vi "AddCurve.vi"(5 "VarPar":string, 7 "CurveName":string, 8 "error in":errorcluster caption="entrée d'erreur (pas d'erreur)", 9 "Y Array":dbl[](array[numeric]), 10 "X Array":dbl[](array[numeric]), 11 "InterfaceIn":refnum<class "Interface.lvclass">) -> (0 "error out":errorcluster caption="sortie d'erreur", 3 "InterfaceOut":refnum<class "Interface.lvclass">)   [LabVIEW 2019, in "Interface.lvclass"]
uses:
  Interface.lvclass
  AddCurveStates.ctl
  CurveSetup.ctl
  Interface.lvclass/Interface.ctl
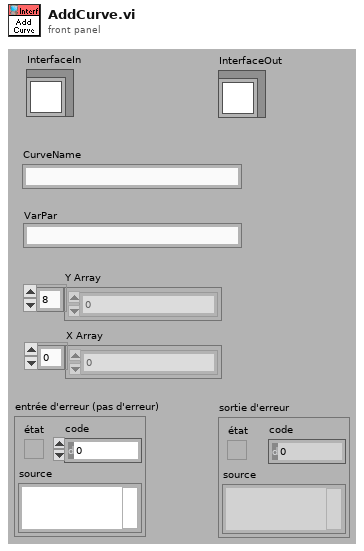
[diagram p1: front panel]
types:
  T1 = typedef "Interface.lvclass/CurveSetup.ctl" = cluster{"CurveName":string, "YParam":string, "XParam":string, "ZParam ":string, "GroupName":string, "LinWdth":u8, "PntCol":u32, "LinCol":u32, "LablFor":u8, "XScale":u32, "YScale":u32, "Interpol":u8, "DisplayName":string, "FillType":i16, "LineStyle":u8, "PntStyle":u8, "BarTyp":u8, "GraphIndex":i32, "Visible":bool, "XScaleName":string, "YScaleName":string, "XYGraph_Ref":refnum<vi>, "Data Only":bool, "DataQ Ref":refnum<queue>, "XParQ Ref":refnum<queue>, "XParamInd":i32, "ScanInd":i32}
  T2 = typedef "AddCurveStates.ctl" = enum16{"CreateCurvePar", "AddToCrvParArr", "CreateDataQ"}
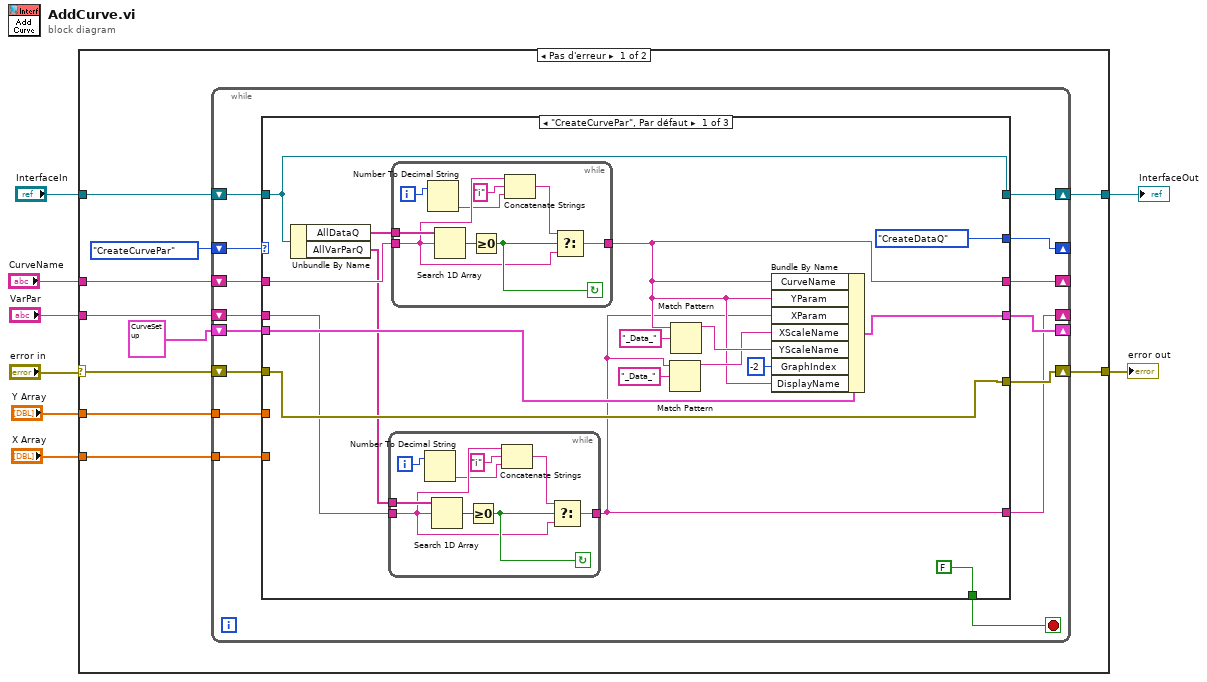
[diagram p0: block diagram]
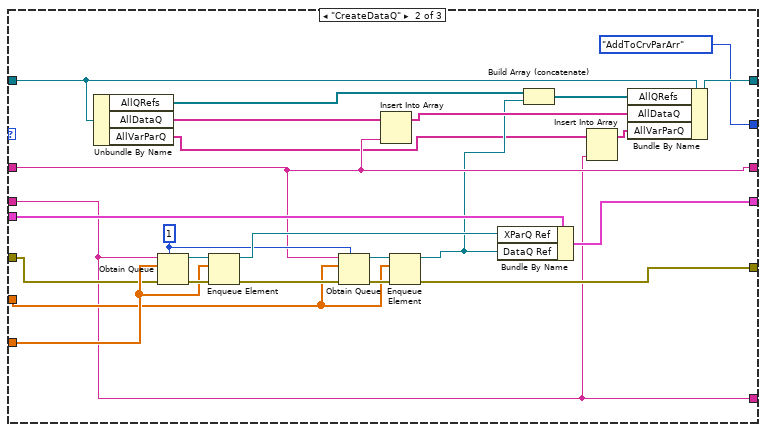
[diagram p2: hidden frame]
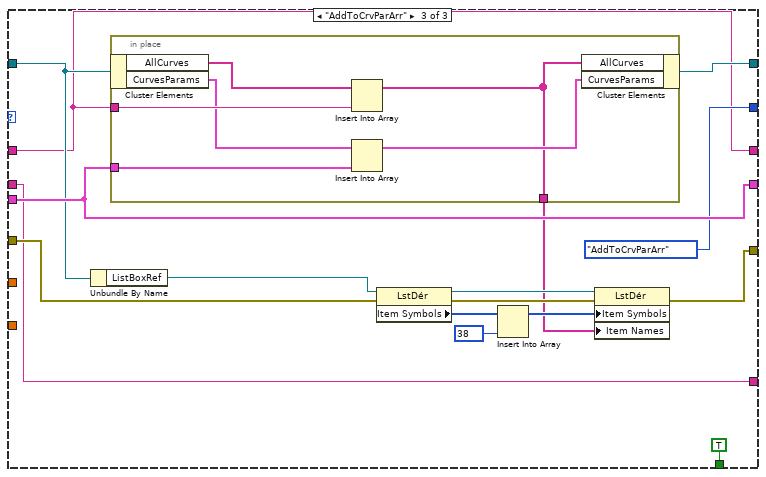
[diagram p3: hidden frame]
diagram:
  n1 = case shown="Pas d'erreur" "error in" {
    selector: "error in" -> [w18 w117]
    tunnel: [w17 w117] -> w7
    tunnel: "CurveName" -> [w15 _]
    tunnel: "VarPar" -> [w12 _]
    tunnel: "InterfaceIn" -> [w13 w116]
    tunnel: [w14 w116] -> w3
    tunnel: "X Array" -> [w10 _]
    tunnel: "Y Array" -> [w9 _]
    frame No Error {
      n2 = while {
        shift-right: [w28] -> w17
        shift-left: w18 -> [w31]
        shift-right: [w29] -> _
        shift-left: AddCurveStates."CreateCurvePar" ("Énum") -> [w32]
        shift-right: [w27] -> w14
        shift-left: w13 -> [w26]
        shift-right: [w25] -> _
        shift-left: T1 {"CurveName"="", "YParam"="", "XParam"="", "ZParam "="", "GroupName"="", "LinWdth"=1, "PntCol"=4294967295, "LinCol"=4294967295, "LablFor"=0, "XScale"=0, "YScale"=0, "Interpol"=2, "DisplayName"="", "FillType"=-1, "LineStyle"=0, "PntStyle"=12, "BarTyp"=0, "GraphIndex"=0, "Visible"=TRUE, "XScaleName"="", "YScaleName"="", "XYGraph_Ref"=refnum, "Data Only"=FALSE, "DataQ Ref"=refnum, "XParQ Ref"=refnum, "XParamInd"=0, "ScanInd"=0} ("CurveParam") -> [w23]
        tunnel: w10 -> [w22]
        tunnel: w9 -> [w21]
        shift-right: [w20] -> _
        shift-left: w15 -> [w30]
        shift-right: [w19] -> _
        shift-left: w12 -> [w24]
        stop <- w33 stop-if-true
        n3 = case shown="\"CreateCurvePar\", Par défaut" w32 {
          tunnel: [FALSE _ TRUE] -> w33
          tunnel: w31 -> [w45 w90 w101]
          tunnel: w30 -> [w38 w76 w94]
          tunnel: w24 -> [w37 w71 w95]
          tunnel: w26 -> [w39 w81 w100]
          tunnel: [AddCurveStates."CreateDataQ" ("Énum") AddCurveStates."AddToCrvParArr" ("Énum") AddCurveStates."AddToCrvParArr" ("Énum")] -> w29
          tunnel: [w45 w85 w97] -> w28
          tunnel: [w39 w80 w109] -> w27
          tunnel: [w47 w83 w108] -> w25
          tunnel: w23 -> [w46 w84 w108]
          tunnel: w22 -> [_ w91 _]
          tunnel: w21 -> [_ w86 _]
          tunnel: [w35 w76 w94] -> w20
          tunnel: [w34 w71 w95] -> w19
          frame "CreateCurvePar", Default {
            n4 = Unbundle By Name(w39) -> ("AllDataQ"=w40:string[], "AllVarParQ"=w36:string[])
            n5 = while {
              tunnel: w36 -> [w68]
              tunnel: w37 -> [w62]
              tunnel: [w66] -> w34
              i -> [w63]
              stop <- w64 continue-if-true
              n6 = Number To Decimal String(number=w63) -> (decimal integer string=w61:string)  [unwired: 1 in]
              n7 = Search 1D Array(1D array=w68, element=w62) -> (index of element=w67:i32)  [unwired: 1 in]
              n8 = Greater Or Equal To 0?(x=w67) -> (x >= 0?=w64:bool)
              n9 = Concatenate Strings(w62, "i" ("chaîne"), w61) -> (w65:string)
              n10 = Select(t=w65, s=w64, f=w62) -> (s? t:f=w66:string)
            }
            n11 = while {
              tunnel: w40 -> [w59]
              tunnel: w38 -> [w53]
              tunnel: [w57] -> w35
              i -> [w54]
              stop <- w55 continue-if-true
              n12 = Number To Decimal String(number=w54) -> (decimal integer string=w52:string)  [unwired: 1 in]
              n13 = Search 1D Array(1D array=w59, element=w53) -> (index of element=w58:i32)  [unwired: 1 in]
              n14 = Greater Or Equal To 0?(x=w58) -> (x >= 0?=w55:bool)
              n15 = Concatenate Strings(w53, "i" ("chaîne"), w52) -> (w56:string)
              n16 = Select(t=w56, s=w55, f=w53) -> (s? t:f=w57:string)
            }
            n17 = Match Pattern(string=w34, regular expression="_Data_" ("expression régulière")) -> (before substring=w41:string)  [unwired: 1 in, 3 out]
            n18 = Match Pattern(string=w35, regular expression="_Data_" ("expression régulière")) -> (before substring=w42:string)  [unwired: 1 in, 3 out]
            n19 = Bundle By Name(cluster=w46, "CurveName"=w35, "YParam"=w35, "XParam"=w34, "XScaleName"=w41, "YScaleName"=w42, "GraphIndex"=-2, "DisplayName"=w35) -> (w47:T1)
          }
          frame "CreateDataQ" {
            w79 = 1 ("max queue size (-1, unlimited)")
            n20 = Unbundle By Name(w81) -> ("AllQRefs"=w73:refnum<queue>[], "AllDataQ"=w77:string[], "AllVarParQ"=w70:string[])
            n21 = Obtain Queue(max queue size (-1, unlimited)=w79, name (unnamed)=w71, element data type=w91, error in (no error)=w90) -> (queue out=w92:refnum<queue>, error out=w93:errorcluster)  [unwired: 1 in, 1 out]
            n22 = Enqueue Element(queue=w92, element=w91, error in (no error)=w93) -> (queue out=w82:refnum<queue>, error out=w87:errorcluster)  [unwired: 1 in, 1 out]
            n23 = Obtain Queue(max queue size (-1, unlimited)=w79, name (unnamed)=w76, element data type=w86, error in (no error)=w87) -> (queue out=w89:refnum<queue>, error out=w88:errorcluster)  [unwired: 1 in, 1 out]
            n24 = Insert Into Array(array=w77, new element=w76) -> (w75:string[])  [unwired: 1 in]
            n25 = Enqueue Element(queue=w89, element=w86, error in (no error)=w88) -> (queue out=w74:refnum<queue>, error out=w85:errorcluster)  [unwired: 1 in, 1 out]
            n26 = Bundle By Name(cluster=w84, "XParQ Ref"=w82, "DataQ Ref"=w74) -> (w83:T1)
            n27 = Build Array (concatenate)(w73, w74) -> (w72:refnum<queue>[])
            n28 = Insert Into Array(array=w70, new element=w71) -> (w69:string[])  [unwired: 1 in]
            n29 = Bundle By Name(cluster=w81, "AllQRefs"=w72, "AllDataQ"=w75, "AllVarParQ"=w69) -> (w80:refnum<class "Interface.lvclass">)
          }
          frame "AddToCrvParArr" {
            n30 = Unbundle By Name(w100) -> ("ListBoxRef"=w99:refnum<vi>)
            n31 = in-place {
              in-place-border: w94 -> [w115]
              in-place-border: w108 -> [w112]
              in-place-border: [w110] -> w98
              n32 = in-place-cluster #1(w100) -> ("AllCurves"=w114:string[], "CurvesParams"=w113:T1[])
              n33 = Insert Into Array(array=w114, new element=w115) -> (w110:string[])  [unwired: 1 in]
              n34 = Insert Into Array(array=w113, new element=w112) -> (w111:T1[])  [unwired: 1 in]
              n35 = in-place-cluster #1("AllCurves"=w110, "CurvesParams"=w111) -> (w109:refnum<class "Interface.lvclass">)
            }
            n36 = property on="Nœud de propriété" class="LstDér"(reference=w99, error in=w101) -> (reference out=w105:refnum<vi>, error out=w106:errorcluster, "Item Symbols"=w104:i32[])
            n37 = Insert Into Array(array=w104, new element=38) -> (w103:i32[])  [unwired: 1 in]
            n38 = property on="Nœud de propriété" class="LstDér"(reference=w105, error in=w106, "Item Symbols"=w103, "Item Names"=w98) -> (error out=w97:errorcluster)  [unwired: 1 out]
          }
        }
      }
    }
    frame Error {
    }
  }
  "error out" <- w7
  "InterfaceOut" <- w3
